vi "Stop Core.vi"(10 "final error code":i32 caption="最终错误代码", 11 "GPS in":refnum<class "GPS.lvclass"> caption="操作者输入") -> (3 "GPS out":refnum<class "GPS.lvclass"> caption="操作者输出")   [LabVIEW 2016, in "GPS.lvlib" / "GPS.lvclass"]
doc: "(<B>Filename</B>: Actor Framework.lvlib:Actor.lvclass:Stop Core.vi)\n\nDefines what the actor does before it stops. Use the <B>final error code</B> input to determine whether the actor shut down in response to an error.\n\nBy default, this method does nothing.子孙类重写该方法，定义出错时的操作，例如，关闭操作者核心方法初始的进程。"
uses:
  GPS.lvclass
  <vilib>/ActorFramework/Actor/Actor.lvclass
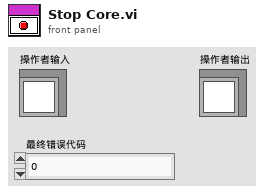
[diagram p1: front panel]
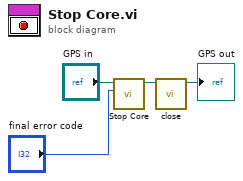
[diagram p0: block diagram]
diagram:
  n1 = call-parent "Stop Core.vi"("final error code"="final error code", "Actor in"="GPS in") -> ("Actor out"=w2:refnum<class "GPS.lvclass">)  [unwired: 9 in]
  n2 = call "close.vi"("GPS 输入"=w2) -> ("GPS 输出"=→"GPS out":refnum<class "GPS.lvclass">)  [unwired: 9 in, 1 out]
